vi "WPI_CameraGet Image From TCP 1.0.0.0.vi"(7 "Camera Mode":u16(ring) items=["Camera Off", "USB Camera SW", "USB Camera HW", "IP Camera"], 8 "error in (no error)":errorcluster, 9 "USB":bool, 10 "Image In":T1, 11 "connection ID":refnum<k5>) -> (0 "error out":errorcluster, 1 "Size":i32, 2 "Image Out":T1, 3 "connection ID out":refnum<k5>)   [LabVIEW 2017]
doc: "Version 1.0.0.0 of the image transfer protocol.\n\nGet the version information first and then gets a raw JPEG string from the TCP connection.\n\nThis software is licensed. Open the labview\\readme\\WPI Robotics Library Open Source License.txt file for more information."
uses:
  <vilib>/vision/Image Controls.llb/IMAQ Image.ctl
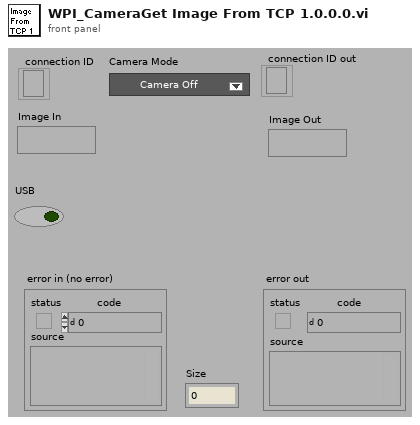
[diagram p1: front panel]
types:
  T1 = typedef "IMAQ Image.ctl" = refnum<image>
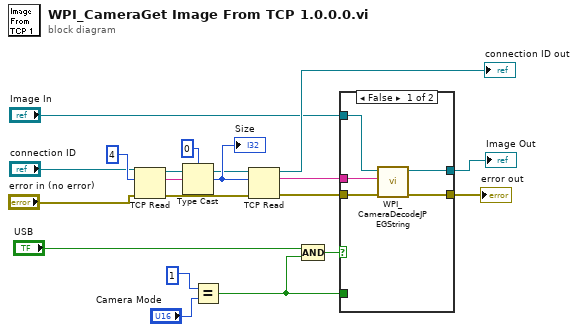
[diagram p0: block diagram]
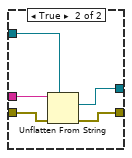
[diagram p2: hidden frame]
diagram:
  n1 = TCP Read(connection ID="connection ID", bytes to read=4, error in (no error)="error in (no error)") -> (connection ID out=w16:refnum<k5>, data out=w17:string, error out=w15:errorcluster)  [unwired: 2 out]
  n2 = Type Cast(type=0 ("bytes to read"), x=w17) -> (*(type *) &x=w19:i32)
  "Size" <- w19
  n3 = Equal?(x=1 ("bytes to read"), y="Camera Mode") -> (x = y?=w3:bool)
  n4 = TCP Read(connection ID=w16, bytes to read=w19, error in (no error)=w15) -> (connection ID out=→"connection ID out":refnum<k5>, data out=w8:string, error out=w6:errorcluster)  [unwired: 2 out]
  n5 = Compound Arithmetic op=AND("USB", w3) -> (w1:bool)
  n6 = case shown="False" w1 {
    tunnel: "Image In" -> [w24 w27]
    tunnel: [w23 w28] -> w10
    tunnel: w8 -> [w22 w29]
    tunnel: [w21 w26] -> w7
    tunnel: w6 -> [w20 w25]
    tunnel: w3 -> [_ _]
    frame False {
      n7 = call <vilib>:"WPI_CameraDecodeJPEGString.vi"("error in"=w20, "Compressed Image"=w22, "Image In"=w24) -> ("error out"=w21:errorcluster, "Image Out"=w23:T1)  [unwired: 3 out]
    }
    frame True {
      n8 = Unflatten From String(type=w27, binary string=w29, error in (no error)=w25) -> (value=w28:T1, error out=w26:errorcluster)  [unwired: 2 in, 1 out]
    }
  }
  "error out" <- w7
  "Image Out" <- w10
